vi "UMLEditor ClipBoard.vi"(1 "menuAction":T1, 2 "SelectedNodes":refnum<class "AbstractNode.lvclass">[](array[class]), 3 "Pos":cluster{dbl, dbl}, 4 "Graph":refnum<class "Graph.lvclass">, 5 "error in (no error)":errorcluster, 7 "LimitPasteToAllowedLocations(True)":bool=TRUE) -> (15 "PastedNodes":refnum<class "AbstractNode.lvclass">[](array[class]), 19 "error out":errorcluster)   [LabVIEW 2014]
doc: "Gets current diagram values"
uses:
  <resource>/Framework/Providers/Open_GDS/UML/UMLEditor/UMLEditor ClipBoardActionType.ctl
  <resource>/Framework/Providers/Open_GDS/UML/AbstractNode_class/AbstractNode.lvclass
  <resource>/Framework/Providers/Open_GDS/UML/Graph_class/Graph.lvclass
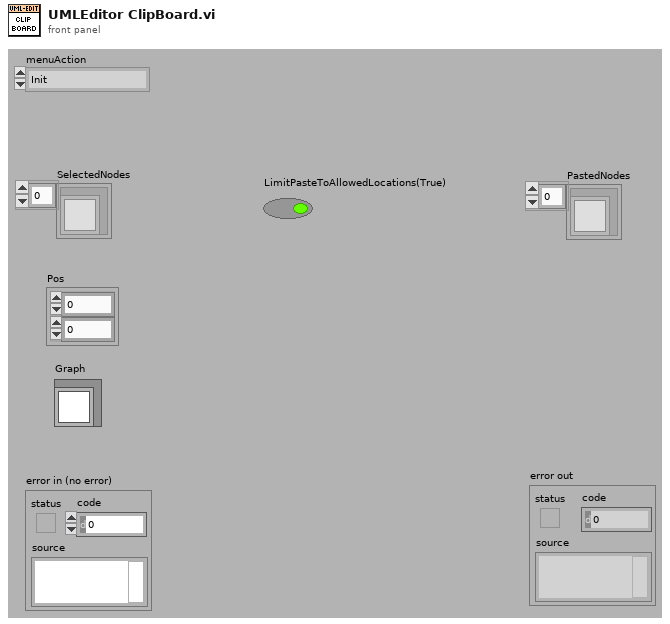
[diagram p1: front panel]
types:
  T1 = typedef "UMLEditor ClipBoardActionType.ctl" = enum16{"Init", "EmptyClipBoard", "InsertToClipBoard", "PasteContentAtPos"}
  T2 = typedef "Rectangle Rectangle2D.ctl" = cluster{"x":dbl, "y":dbl, "width":dbl, "height":dbl}
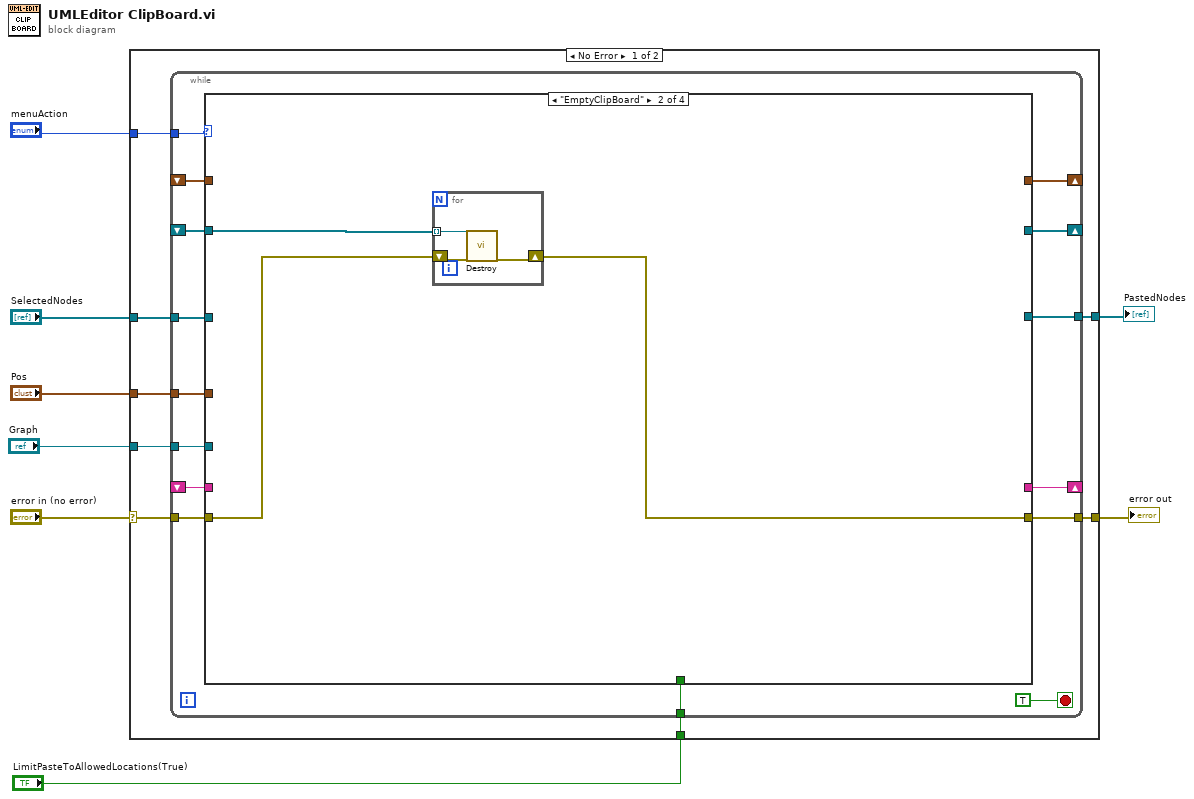
[diagram p0: block diagram]
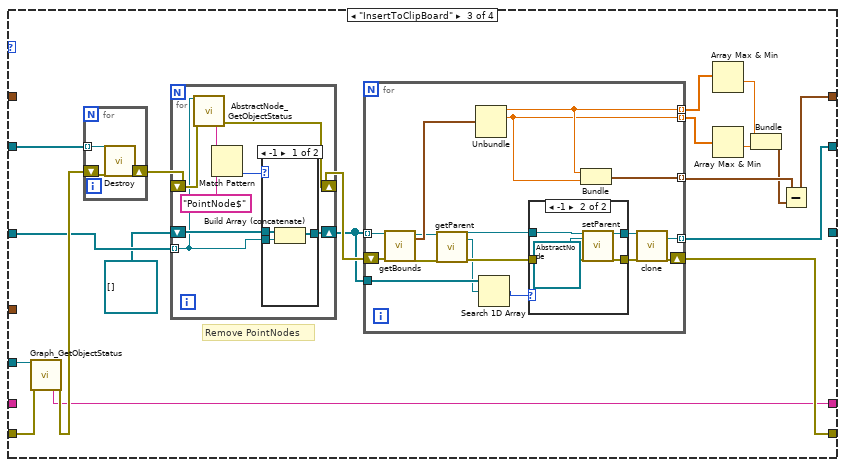
[diagram p3: hidden frame]
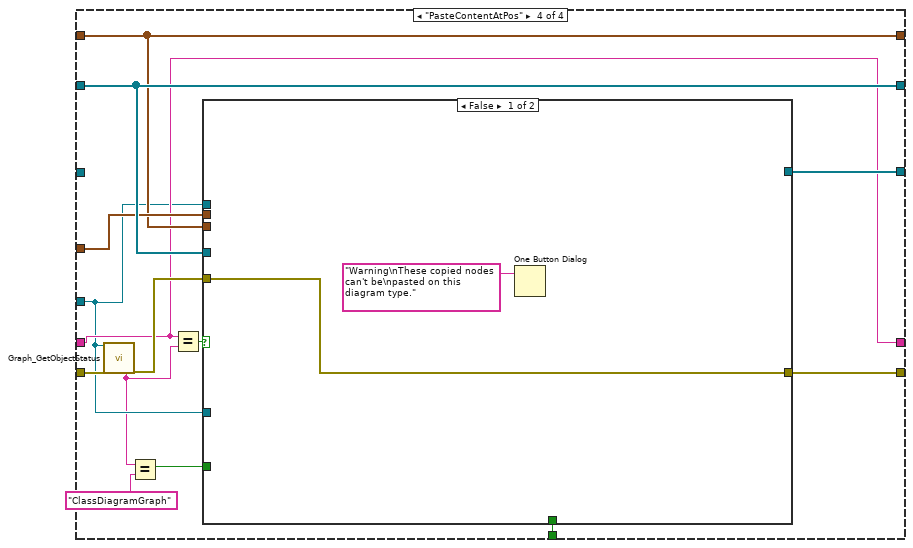
[diagram p6: hidden frame]
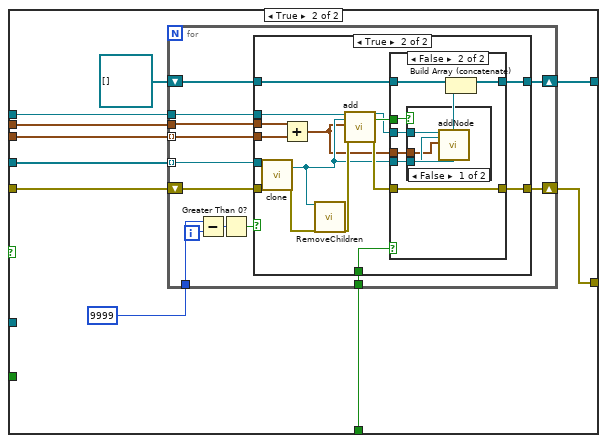
[diagram p7: hidden frame]
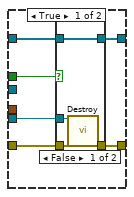
[diagram p9: hidden frame]
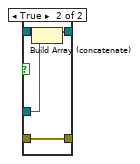
[diagram p10: hidden frame]
diagram:
  n1 = case shown="No Error" "error in (no error)" {
    selector: "error in (no error)" -> [w14 w178]
    tunnel: [w15 w178] -> w7
    tunnel: "menuAction" -> [w16 _]
    tunnel: "SelectedNodes" -> [w13 _]
    tunnel: "Pos" -> [w12 _]
    tunnel: "Graph" -> [w11 _]
    tunnel: [w10 _] -> w2
    tunnel: "LimitPasteToAllowedLocations(True)" -> [w9 _]
    frame No Error {
      n2 = while {
        tunnel: w16 -> [w30]
        tunnel: [w28] -> w15
        tunnel: w14 -> [w29]
        tunnel: w13 -> [w27]
        shift-right: [w26] -> _
        shift-left: _ -> [w25]
        tunnel: w12 -> [w24]
        tunnel: w11 -> [w23]
        tunnel: [w22] -> w10
        shift-right: [w21] -> _
        shift-left: _ -> [w20]
        shift-right: [w19] -> _
        shift-left: _ -> [w18]
        tunnel: w9 -> [w17]
        stop <- TRUE stop-if-true
        n3 = case shown="\"EmptyClipBoard\"" w30 {
          tunnel: w29 -> [w32 w34 w46 w105]
          tunnel: [w32 w33 w57 w108] -> w28
          tunnel: w27 -> [_ _ w43 _]
          tunnel: [_ _ w56 w110] -> w26
          tunnel: w25 -> [_ w35 w55 w110]
          tunnel: w24 -> [_ _ _ w109]
          tunnel: w23 -> [_ _ w47 w101]
          tunnel: [_ _ _ w107] -> w22
          tunnel: [_ _ w48 w106] -> w21
          tunnel: w20 -> [_ _ _ w106]
          tunnel: [_ _ w44 w102] -> w19
          tunnel: w18 -> [_ _ _ w102]
          tunnel: w17 -> [_ _ _ w97]
          frame "Init", Default {
          }
          frame "EmptyClipBoard" {
            n4 = for {
              tunnel: w35 -> [w38] mode=indexing
              shift-right: [w36] -> w33
              shift-left: w34 -> [w37]
              n5 = call-dynamic "Destroy.vi"("reference"=w38, "error in (no error)"=w37) -> ("error out"=w36:errorcluster)  [unwired: 16 in, 1 out]
            }
          }
          frame "InsertToClipBoard" {
            # "Remove PointNodes"
            n6 = call <resource>:"Graph_GetObjectStatus.vi"("reference in"=w47, "error in (no error)"=w46) -> ("Class name"=w44:string, "error out"=w45:errorcluster)  [unwired: 16 out]
            n7 = for {
              tunnel: w55 -> [w72] mode=indexing
              shift-right: [w70] -> w42
              shift-left: w45 -> [w71]
              n8 = call-dynamic "Destroy.vi"("reference"=w72, "error in (no error)"=w71) -> ("error out"=w70:errorcluster)  [unwired: 16 in, 1 out]
            }
            n9 = for {
              tunnel: w43 -> [w59] mode=indexing
              shift-right: [w58] -> w41
              shift-left: w42 -> [w62]
              shift-right: [w60] -> w39
              shift-left: refnum<class "AbstractNode.lvclass">[] [] -> [w61]
              n10 = call <resource>:"AbstractNode_GetObjectStatus.vi"("reference in"=w59, "error in (no error)"=w62) -> ("Class name"=w65:string, "error out"=w58:errorcluster)  [unwired: 16 out]
              n11 = Match Pattern(string=w65, regular expression="PointNode$") -> (offset past match=w63:i32)  [unwired: 4 out]
              n12 = case shown="-1" w63 {
                tunnel: w61 -> [w68 w69]
                tunnel: w59 -> [w67 _]
                tunnel: [w66 w69] -> w60
                frame -1 {
                  n13 = Build Array (concatenate)(w68, w67) -> (w66:refnum<class "AbstractNode.lvclass">[])
                }
                frame Default {
                }
              }
            }
            n14 = for {
              tunnel: w39 -> [w87] mode=indexing
              shift-right: [w89] -> w57
              shift-left: w41 -> [w86]
              tunnel: [w88] -> w56 mode=indexing
              tunnel: [w82] -> w52 mode=indexing
              tunnel: [w84] -> w54 mode=indexing
              tunnel: [w83] -> w53 mode=indexing
              tunnel: w39 -> [w76]
              n15 = call-dynamic "getBounds.vi"("reference"=w87, "error in (no error)"=w86) -> ("reference out"=w81:refnum<class "AbstractNode.lvclass">, "bounds"=w85:T2, "error out"=w80:errorcluster)  [unwired: 15 in]
              n16 = call-dynamic "getParent.vi"("reference"=w81, "error in (no error)"=w80) -> ("reference out"=w75:refnum<class "AbstractNode.lvclass">, "parentNode"=w74:refnum<class "AbstractNode.lvclass">, "error out"=w77:errorcluster)  [unwired: 13 in, 2 out]
              n17 = Unbundle(w85) -> ("x"=w84:dbl, "y"=w83:dbl)  [unwired: 2 out]
              n18 = Search 1D Array(1D array=w76, element=w74) -> (index of element=w73:i32)  [unwired: 1 in]
              n19 = case shown="-1" w73 {
                tunnel: w75 -> [w90 w96]
                tunnel: [w90 w95] -> w79
                tunnel: [w91 w94] -> w78
                tunnel: w77 -> [w91 w93]
                frame 0, Default {
                }
                frame -1 {
                  n20 = call-dynamic "setParent.vi"("reference"=w96, "node"=refnum<class "AbstractNode.lvclass"> refnum, "error in (no error)"=w93) -> ("reference out"=w95:refnum<class "AbstractNode.lvclass">, "error out"=w94:errorcluster)  [unwired: 15 in]
                }
              }
              n21 = Bundle("x"=w84, "y"=w83) -> (w82:cluster{"x":dbl, "y":dbl})  [unwired: 1 out]
              n22 = call-dynamic "clone.vi"("reference"=w79, "error in (no error)"=w78) -> ("clonedAbstractNode"=w88:refnum<class "AbstractNode.lvclass">, "error out"=w89:errorcluster)  [unwired: 15 in, 1 out]
            }
            n23 = Array Max & Min(array=w54) -> (min value=w50:dbl)  [unwired: 3 out]
            n24 = Array Max & Min(array=w53) -> (min value=w51:dbl)  [unwired: 3 out]
            n25 = Bundle(w50, w51) -> (w49:cluster{dbl, dbl})  [unwired: 1 out]
            n26 = Subtract(x=w52, y=w49) -> (x-y=w48:cluster{dbl, dbl}[])
          }
          frame "PasteContentAtPos" {
            n27 = call <resource>:"Graph_GetObjectStatus.vi"("reference in"=w101, "error in (no error)"=w105) -> ("Class name"=w100:string, "error out"=w104:errorcluster)  [unwired: 16 out]
            n28 = Equal?(x=w100, y="ClassDiagramGraph") -> (x = y?=w98:bool)
            n29 = Equal?(x=w102, y=w100) -> (x = y?=w103:bool)
            n30 = case shown="False" w103 {
              tunnel: w110 -> [_ w122]
              tunnel: w109 -> [_ w121]
              tunnel: [w111 w120] -> w108
              tunnel: [_ w118] -> w107
              tunnel: w106 -> [_ w117]
              tunnel: w104 -> [w111 w116]
              tunnel: w101 -> [_ w115]
              tunnel: w101 -> [_ _]
              tunnel: w98 -> [_ _]
              tunnel: w97 -> [_ w113]
              frame False {
                n31 = One Button Dialog(message="Warning\nThese copied nodes can't be\npasted on this diagram type.") -> ()  [unwired: 2 out]
              }
              frame True {
                n32 = for {
                  tunnel: w122 -> [w135] mode=indexing
                  shift-right: [w133] -> w120
                  shift-left: w116 -> [w134]
                  tunnel: w121 -> [w129]
                  tunnel: w115 -> [w132]
                  shift-right: [w130] -> w118
                  shift-left: refnum<class "AbstractNode.lvclass">[] [] -> [w131]
                  tunnel: w117 -> [w128] mode=indexing
                  tunnel: i16 9999 -> [w127]
                  tunnel: w113 -> [w123]
                  i -> [w126]
                  n33 = Subtract(x=w127, y=w126) -> (x-y=w125:i32)
                  n34 = Greater Than 0?(x=w125) -> (x > 0?=w124:bool)
                  n35 = case shown="True" w124 {
                    tunnel: w135 -> [_ w152]
                    tunnel: w134 -> [w137 w151]
                    tunnel: [w137 w150] -> w133
                    tunnel: w132 -> [_ w149]
                    tunnel: w131 -> [w136 w148]
                    tunnel: [w136 w147] -> w130
                    tunnel: w129 -> [_ w146]
                    tunnel: w128 -> [_ w145]
                    tunnel: w123 -> [_ w140]
                    frame False {
                    }
                    frame True {
                      n36 = call-dynamic "clone.vi"("reference"=w152, "error in (no error)"=w151) -> ("clonedAbstractNode"=w142:refnum<class "AbstractNode.lvclass">, "error out"=w144:errorcluster)  [unwired: 15 in, 1 out]
                      n37 = Add(x=w146, y=w145) -> (x+y=w138:cluster{dbl, dbl})
                      n38 = call-dynamic "RemoveChildren.vi"("reference"=w142, "error in (no error)"=w144) -> ("error out"=w143:errorcluster)  [unwired: 15 in, 2 out]
                      n39 = call-dynamic "add.vi"("reference"=w149, "node"=w142, "point"=w138, "error in (no error)"=w143) -> ("reference out"=w139:refnum<class "Graph.lvclass">, "added"=w141:bool, "error out"=w153:errorcluster)  [unwired: 13 in]
                      n40 = case shown="False" w140 {
                        tunnel: w153 -> [w159 w174]
                        tunnel: [w158 w174] -> w150
                        tunnel: w148 -> [w157 w173]
                        tunnel: [w156 w172] -> w147
                        tunnel: w142 -> [w155 w169]
                        tunnel: w141 -> [w154 w171]
                        tunnel: w139 -> [_ w170]
                        tunnel: w138 -> [_ w168]
                        frame True {
                          n41 = case shown="False" w154 {
                            tunnel: w159 -> [w163 w167]
                            tunnel: [w162 w167] -> w158
                            tunnel: w155 -> [w161 w165]
                            tunnel: w157 -> [w160 w166]
                            tunnel: [w160 w164] -> w156
                            frame False {
                              n42 = call-dynamic "Destroy.vi"("reference"=w161, "error in (no error)"=w163) -> ("error out"=w162:errorcluster)  [unwired: 16 in, 1 out]
                            }
                            frame True {
                              n43 = Build Array (concatenate)(w166, w165) -> (w164:refnum<class "AbstractNode.lvclass">[])
                            }
                          }
                        }
                        frame False {
                          n44 = case shown="False" w171 {
                            tunnel: w170 -> [w177 _]
                            tunnel: w169 -> [w176 _]
                            tunnel: w168 -> [w175 _]
                            frame False {
                              n45 = call-dynamic "addNode.vi"("reference"=w177, "node"=w176, "point"=w175) -> ()  [unwired: 15 in, 2 out]
                            }
                            frame True {
                            }
                          }
                          n46 = Build Array (concatenate)(w173, w169) -> (w172:refnum<class "AbstractNode.lvclass">[])
                        }
                      }
                    }
                  }
                }
              }
            }
          }
        }
      }
    }
    frame Error {
    }
  }
  "error out" <- w7
  "PastedNodes" <- w2
